vi "MainFrame5.vi"() -> ()   [LabVIEW 2014]
doc: "This example demonstrates the easiest method of inserting a VI into a subpanel"
uses:
  typedef controls/test mainframe bottons.ctl
panel:
  in  "Cluster":T1
  out "panel?":u8=2
  # "Mainframe Test Program"
  # "your application name"
  # "version 5.0"
  # "F3"
  # "F4"
  # "F5"
  # "F6"
  # "F7"
  # "F8"
  # "F9"
  # "F10"
  # "F12"
  # "version 1.5"
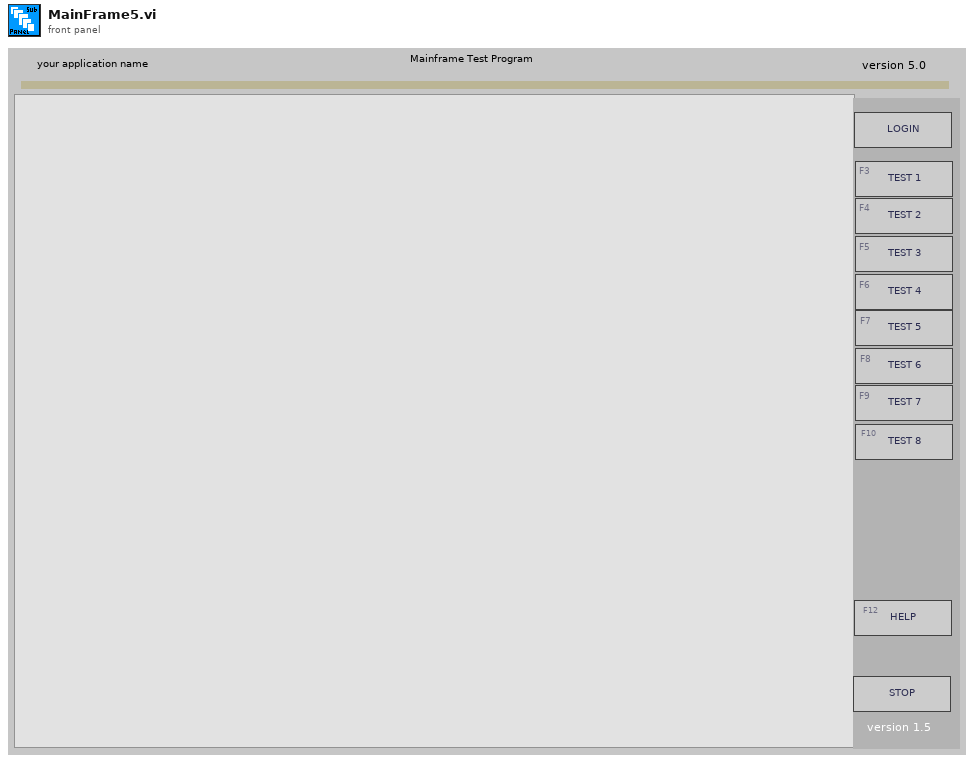
[diagram p1: front panel]
types:
  T1 = typedef "test mainframe bottons.ctl" = cluster{"LOGIN":bool, "TEST 1":bool, "TEST 2":bool, "TEST 3":bool, "TEST 4":bool, "TEST 5":bool, "TEST 6":bool, "TEST 7":bool, "TEST 8":bool, "HELP":bool, "STOP":bool}
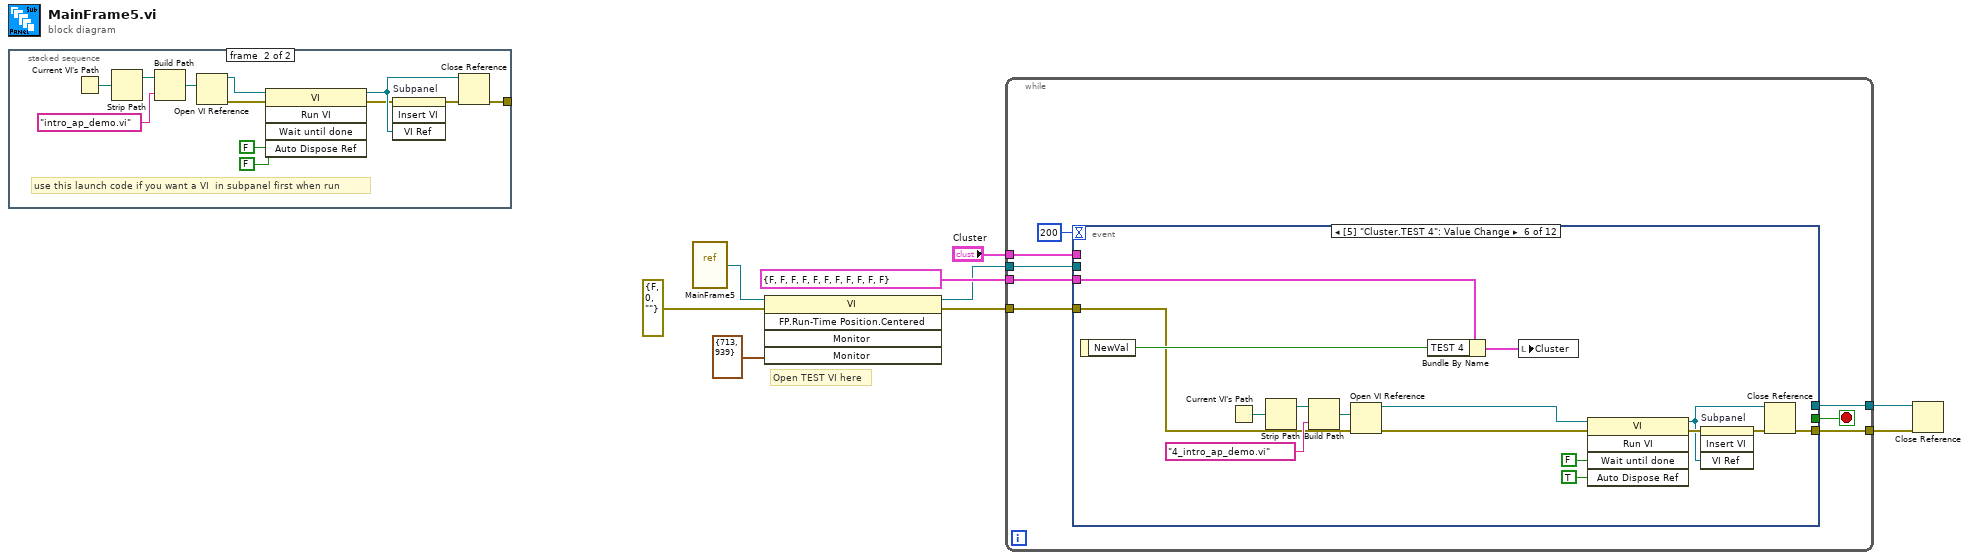
[diagram p0: block diagram]
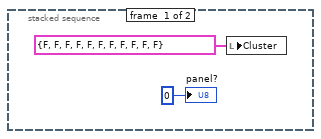
[diagram p2: hidden frame]
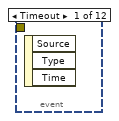
[diagram p3: hidden frame]
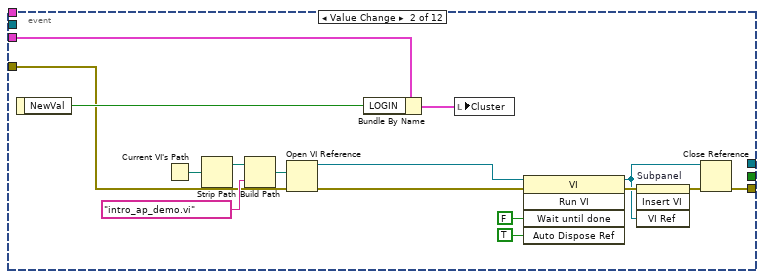
[diagram p4: hidden frame]
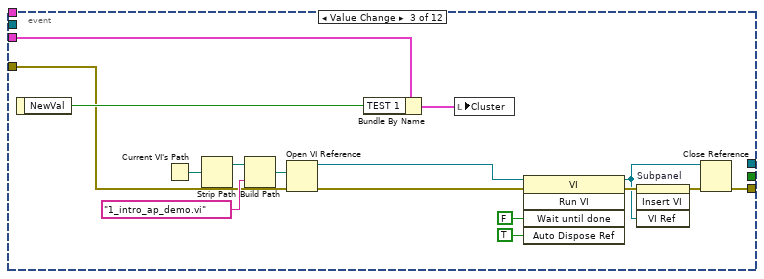
[diagram p5: hidden frame]
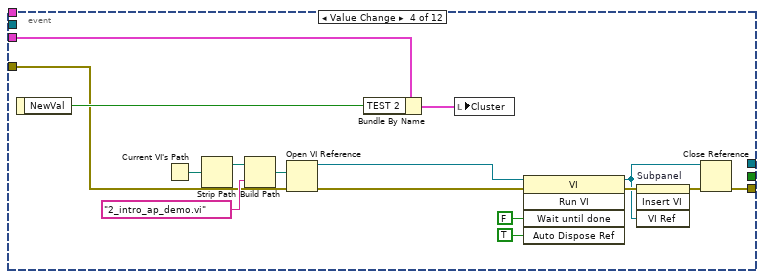
[diagram p6: hidden frame]
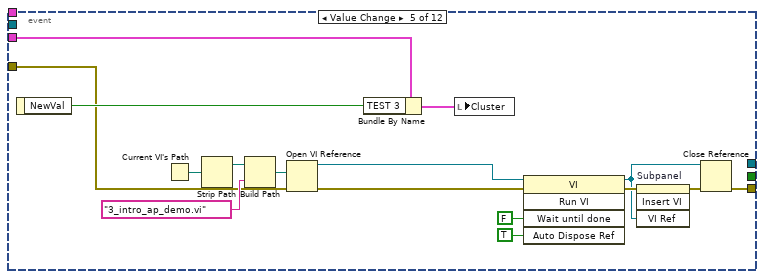
[diagram p7: hidden frame]
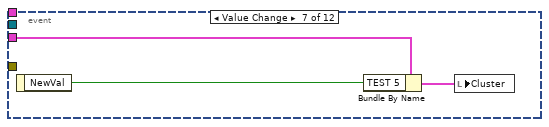
[diagram p8: hidden frame]
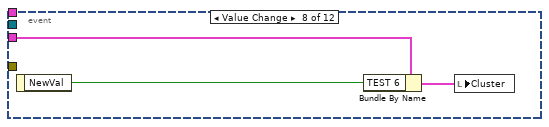
[diagram p9: hidden frame]
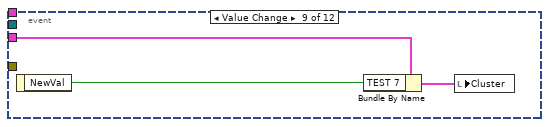
[diagram p10: hidden frame]
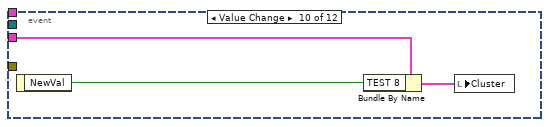
[diagram p11: hidden frame]
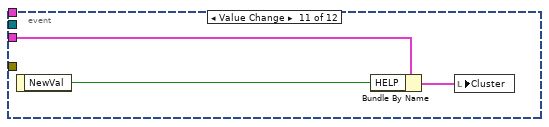
[diagram p12: hidden frame]
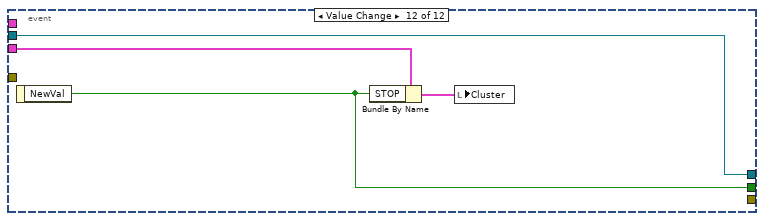
[diagram p13: hidden frame]
diagram:
  # "Open TEST VI here"
  n1 = stacked-sequence {
    tunnel: [_ w12] -> _
    frame #0 {
      n2 = local write "Cluster"(T1 {"LOGIN"=FALSE, "TEST 1"=FALSE, "TEST 2"=FALSE, "TEST 3"=FALSE, "TEST 4"=FALSE, "TEST 5"=FALSE, "TEST 6"=FALSE, "TEST 7"=FALSE, "TEST 8"=FALSE, "HELP"=FALSE, "STOP"=FALSE} ("Cluster")) -> ()
      "panel?" <- u8 0 ("Disabled")
    }
    frame #1 {
      # "use this launch code if you want a VI  in subpanel first when run"
      n3 = Current VI's Path() -> (path=w18:path)
      n4 = Strip Path(path=w18) -> (stripped path=w17:path)  [unwired: 1 out]
      n5 = Build Path(base path=w17, name or relative path="intro_ap_demo.vi") -> (appended path=w21:path)
      n6 = Open VI Reference(vi path=w21) -> (vi reference=w22:refnum<vi>, error out=w23:errorcluster)  [unwired: 5 in]
      n7 = invoke class="VI" method="Run VI"(reference=w22, error in=w23, "Wait until done"=FALSE, "Auto Dispose Ref"=FALSE ("Wait until done")) -> (reference out=w14:refnum<vi>, error out=w13:errorcluster)  [unwired: 1 in, 3 out]
      n8 = invoke on="Subpanel" class="SubPnl" method="Insert VI"(error in=w13, "VI Ref"=w14) -> (error out=w15:errorcluster)  [unwired: 2 in, 3 out]
      n9 = Close Reference(reference=w14, error in (no error)=w15) -> (error out=w12:errorcluster)
    }
  }
  n10 = vi-ref "MainFrame5.vi"() -> (w8:refnum<vi>)
  n11 = invoke class="VI" method="FP.Run-Time Position.Centered"(reference=w8, error in=errorcluster {"status"=FALSE, "code"=0, "source"=""} ("error in (no error)"), "Monitor"=cluster{"Height":i16, "Width":i16} {"Height"=713, "Width"=939} ("Size")) -> (reference out=w2:refnum<vi>, error out=w7:errorcluster)  [unwired: 2 in, 3 out]
  n12 = while {
    tunnel: "Cluster" -> [w30]
    tunnel: [w28] -> w3
    tunnel: w7 -> [w27]
    tunnel: T1 {"LOGIN"=FALSE, "TEST 1"=FALSE, "TEST 2"=FALSE, "TEST 3"=FALSE, "TEST 4"=FALSE, "TEST 5"=FALSE, "TEST 6"=FALSE, "TEST 7"=FALSE, "TEST 8"=FALSE, "HELP"=FALSE, "STOP"=FALSE} ("Cluster") -> [w26]
    tunnel: w2 -> [w25]
    tunnel: [w24] -> w1
    stop <- w29 stop-if-true
    n13 = event shown="[5] \"Cluster.TEST 4\": Value Change" {
      selector: _ -> [_ _ _ _ _ _ _ _ _ _ _ _]
      dyn-events: _ -> [_ _ _ _ _ _ _ _ _ _ _ _]
      timeout: 200 -> [_ _ _ _ _ _ _ _ _ _ _ _]
      tunnel: [_ _ _ _ _ _ _ _ _ _ _ w130] -> w29
      tunnel: w30 -> [_ _ _ _ _ _ _ _ _ _ _ _]
      tunnel: [_ w36 w63 w79 w95 w111 _ _ _ _ _ _] -> w28
      tunnel: w27 -> [_ w33 w50 w66 w82 w98 _ _ _ _ _ _]
      tunnel: w26 -> [_ w32 w49 w65 w81 w97 w113 w116 w119 w122 w125 w129]
      tunnel: w25 -> [_ _ _ _ _ _ _ _ _ _ _ w127]
      tunnel: [_ _ _ _ _ _ _ _ _ _ _ w127] -> w24
      event Timeout {
        n14 = event-data() -> ()  [unwired: 1 in, 3 out]
      }
      event Value Change {
        n15 = event-data() -> ("NewVal"=w34:bool)  [unwired: 1 in]
        n16 = Current VI's Path() -> (path=w43:path)
        n17 = Strip Path(path=w43) -> (stripped path=w45:path)  [unwired: 1 out]
        n18 = Build Path(base path=w45, name or relative path="intro_ap_demo.vi") -> (appended path=w44:path)
        n19 = Open VI Reference(vi path=w44, error in (no error)=w33) -> (vi reference=w38:refnum<vi>, error out=w42:errorcluster)  [unwired: 4 in]
        n20 = Bundle By Name(cluster=w32, "LOGIN"=w34) -> (w35:T1)
        n21 = local write "Cluster"(w35) -> ()
        n22 = invoke class="VI" method="Run VI"(reference=w38, error in=w42, "Wait until done"=FALSE, "Auto Dispose Ref"=TRUE ("Wait until done")) -> (reference out=w37:refnum<vi>, error out=w47:errorcluster)  [unwired: 1 in, 3 out]
        n23 = invoke on="Subpanel" class="SubPnl" method="Insert VI"(error in=w47, "VI Ref"=w37) -> (error out=w46:errorcluster)  [unwired: 2 in, 3 out]
        n24 = Close Reference(reference=w37, error in (no error)=w46) -> (error out=w36:errorcluster)
      }
      event Value Change {
        n25 = event-data() -> ("NewVal"=w62:bool)  [unwired: 1 in]
        n26 = Current VI's Path() -> (path=w57:path)
        n27 = Strip Path(path=w57) -> (stripped path=w59:path)  [unwired: 1 out]
        n28 = Build Path(base path=w59, name or relative path="1_intro_ap_demo.vi") -> (appended path=w58:path)
        n29 = Open VI Reference(vi path=w58, error in (no error)=w50) -> (vi reference=w53:refnum<vi>, error out=w56:errorcluster)  [unwired: 4 in]
        n30 = Bundle By Name(cluster=w49, "TEST 1"=w62) -> (w48:T1)
        n31 = local write "Cluster"(w48) -> ()
        n32 = invoke class="VI" method="Run VI"(reference=w53, error in=w56, "Wait until done"=FALSE, "Auto Dispose Ref"=TRUE ("Wait until done")) -> (reference out=w52:refnum<vi>, error out=w61:errorcluster)  [unwired: 1 in, 3 out]
        n33 = invoke on="Subpanel" class="SubPnl" method="Insert VI"(error in=w61, "VI Ref"=w52) -> (error out=w60:errorcluster)  [unwired: 2 in, 3 out]
        n34 = Close Reference(reference=w52, error in (no error)=w60) -> (error out=w63:errorcluster)
      }
      event Value Change {
        n35 = event-data() -> ("NewVal"=w78:bool)  [unwired: 1 in]
        n36 = Current VI's Path() -> (path=w73:path)
        n37 = Strip Path(path=w73) -> (stripped path=w75:path)  [unwired: 1 out]
        n38 = Build Path(base path=w75, name or relative path="2_intro_ap_demo.vi") -> (appended path=w74:path)
        n39 = Open VI Reference(vi path=w74, error in (no error)=w66) -> (vi reference=w69:refnum<vi>, error out=w72:errorcluster)  [unwired: 4 in]
        n40 = Bundle By Name(cluster=w65, "TEST 2"=w78) -> (w64:T1)
        n41 = local write "Cluster"(w64) -> ()
        n42 = invoke class="VI" method="Run VI"(reference=w69, error in=w72, "Wait until done"=FALSE, "Auto Dispose Ref"=TRUE ("Wait until done")) -> (reference out=w68:refnum<vi>, error out=w77:errorcluster)  [unwired: 1 in, 3 out]
        n43 = invoke on="Subpanel" class="SubPnl" method="Insert VI"(error in=w77, "VI Ref"=w68) -> (error out=w76:errorcluster)  [unwired: 2 in, 3 out]
        n44 = Close Reference(reference=w68, error in (no error)=w76) -> (error out=w79:errorcluster)
      }
      event Value Change {
        n45 = event-data() -> ("NewVal"=w94:bool)  [unwired: 1 in]
        n46 = Current VI's Path() -> (path=w89:path)
        n47 = Strip Path(path=w89) -> (stripped path=w91:path)  [unwired: 1 out]
        n48 = Build Path(base path=w91, name or relative path="3_intro_ap_demo.vi") -> (appended path=w90:path)
        n49 = Open VI Reference(vi path=w90, error in (no error)=w82) -> (vi reference=w85:refnum<vi>, error out=w88:errorcluster)  [unwired: 4 in]
        n50 = Bundle By Name(cluster=w81, "TEST 3"=w94) -> (w80:T1)
        n51 = local write "Cluster"(w80) -> ()
        n52 = invoke class="VI" method="Run VI"(reference=w85, error in=w88, "Wait until done"=FALSE, "Auto Dispose Ref"=TRUE ("Wait until done")) -> (reference out=w84:refnum<vi>, error out=w93:errorcluster)  [unwired: 1 in, 3 out]
        n53 = invoke on="Subpanel" class="SubPnl" method="Insert VI"(error in=w93, "VI Ref"=w84) -> (error out=w92:errorcluster)  [unwired: 2 in, 3 out]
        n54 = Close Reference(reference=w84, error in (no error)=w92) -> (error out=w95:errorcluster)
      }
      event Value Change {
        n55 = event-data() -> ("NewVal"=w110:bool)  [unwired: 1 in]
        n56 = Current VI's Path() -> (path=w105:path)
        n57 = Strip Path(path=w105) -> (stripped path=w107:path)  [unwired: 1 out]
        n58 = Build Path(base path=w107, name or relative path="4_intro_ap_demo.vi") -> (appended path=w106:path)
        n59 = Open VI Reference(vi path=w106, error in (no error)=w98) -> (vi reference=w101:refnum<vi>, error out=w104:errorcluster)  [unwired: 4 in]
        n60 = Bundle By Name(cluster=w97, "TEST 4"=w110) -> (w96:T1)
        n61 = local write "Cluster"(w96) -> ()
        n62 = invoke class="VI" method="Run VI"(reference=w101, error in=w104, "Wait until done"=FALSE, "Auto Dispose Ref"=TRUE ("Wait until done")) -> (reference out=w100:refnum<vi>, error out=w109:errorcluster)  [unwired: 1 in, 3 out]
        n63 = invoke on="Subpanel" class="SubPnl" method="Insert VI"(error in=w109, "VI Ref"=w100) -> (error out=w108:errorcluster)  [unwired: 2 in, 3 out]
        n64 = Close Reference(reference=w100, error in (no error)=w108) -> (error out=w111:errorcluster)
      }
      event Value Change {
        n65 = event-data() -> ("NewVal"=w114:bool)  [unwired: 1 in]
        n66 = Bundle By Name(cluster=w113, "TEST 5"=w114) -> (w112:T1)
        n67 = local write "Cluster"(w112) -> ()
      }
      event Value Change {
        n68 = event-data() -> ("NewVal"=w117:bool)  [unwired: 1 in]
        n69 = Bundle By Name(cluster=w116, "TEST 6"=w117) -> (w115:T1)
        n70 = local write "Cluster"(w115) -> ()
      }
      event Value Change {
        n71 = event-data() -> ("NewVal"=w120:bool)  [unwired: 1 in]
        n72 = Bundle By Name(cluster=w119, "TEST 7"=w120) -> (w118:T1)
        n73 = local write "Cluster"(w118) -> ()
      }
      event Value Change {
        n74 = event-data() -> ("NewVal"=w123:bool)  [unwired: 1 in]
        n75 = Bundle By Name(cluster=w122, "TEST 8"=w123) -> (w121:T1)
        n76 = local write "Cluster"(w121) -> ()
      }
      event Value Change {
        n77 = event-data() -> ("NewVal"=w126:bool)  [unwired: 1 in]
        n78 = Bundle By Name(cluster=w125, "HELP"=w126) -> (w124:T1)
        n79 = local write "Cluster"(w124) -> ()
      }
      event Value Change {
        n80 = event-data() -> ("NewVal"=w130:bool)  [unwired: 1 in]
        n81 = Bundle By Name(cluster=w129, "STOP"=w130) -> (w128:T1)
        n82 = local write "Cluster"(w128) -> ()
      }
    }
  }
  n83 = Close Reference(reference=w1, error in (no error)=w3) -> ()  [unwired: 1 out]
